vi "Convert Waveform to Data.vi"(0 "Waveform Graph":digitalwaveform(graph), 1 "Register":u8=28 format="%.0x", 2 "Ext_Read_Num_Reg":u8) -> (4 "Converted Data":T1 {"Register" max=31 format="%.0x"; "Slave Address" max=15 format="%.0x"}, 6 "Ext_Read_Reg":i32[](array[numeric]), 8 "Ext_Read_Data":u8[](array[numeric]))   [LabVIEW 2013]
uses:
  <vilib>/Waveform/DTblOps.llb/DTbl Digital to Boolean Array.vi
panel:
  # "i"
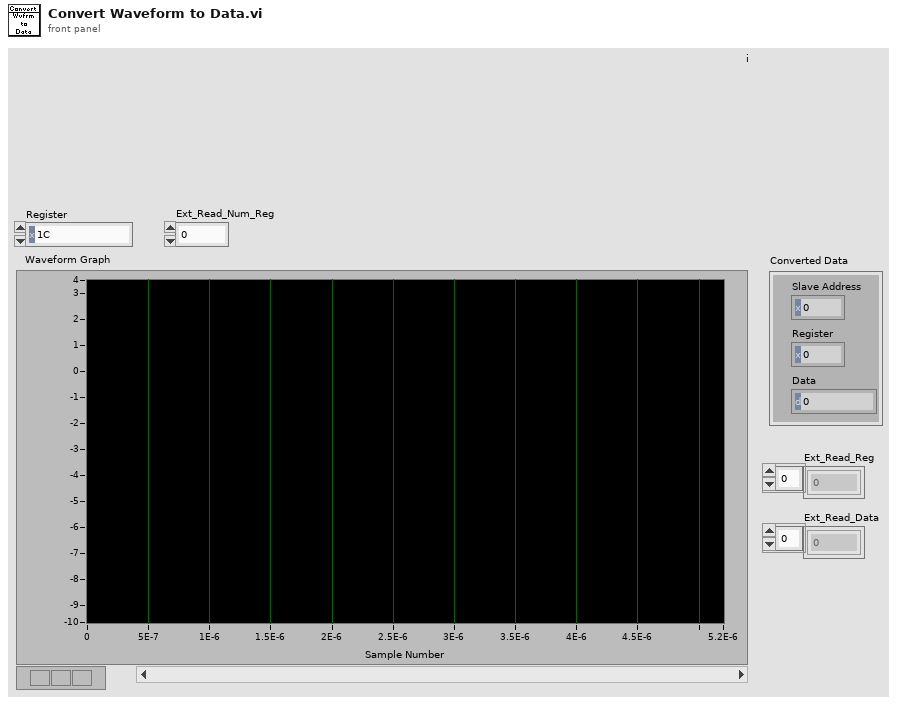
[diagram p1: front panel]
types:
  T1 = cluster{"Slave Address":u8, "Register":u8, "Data":u8}
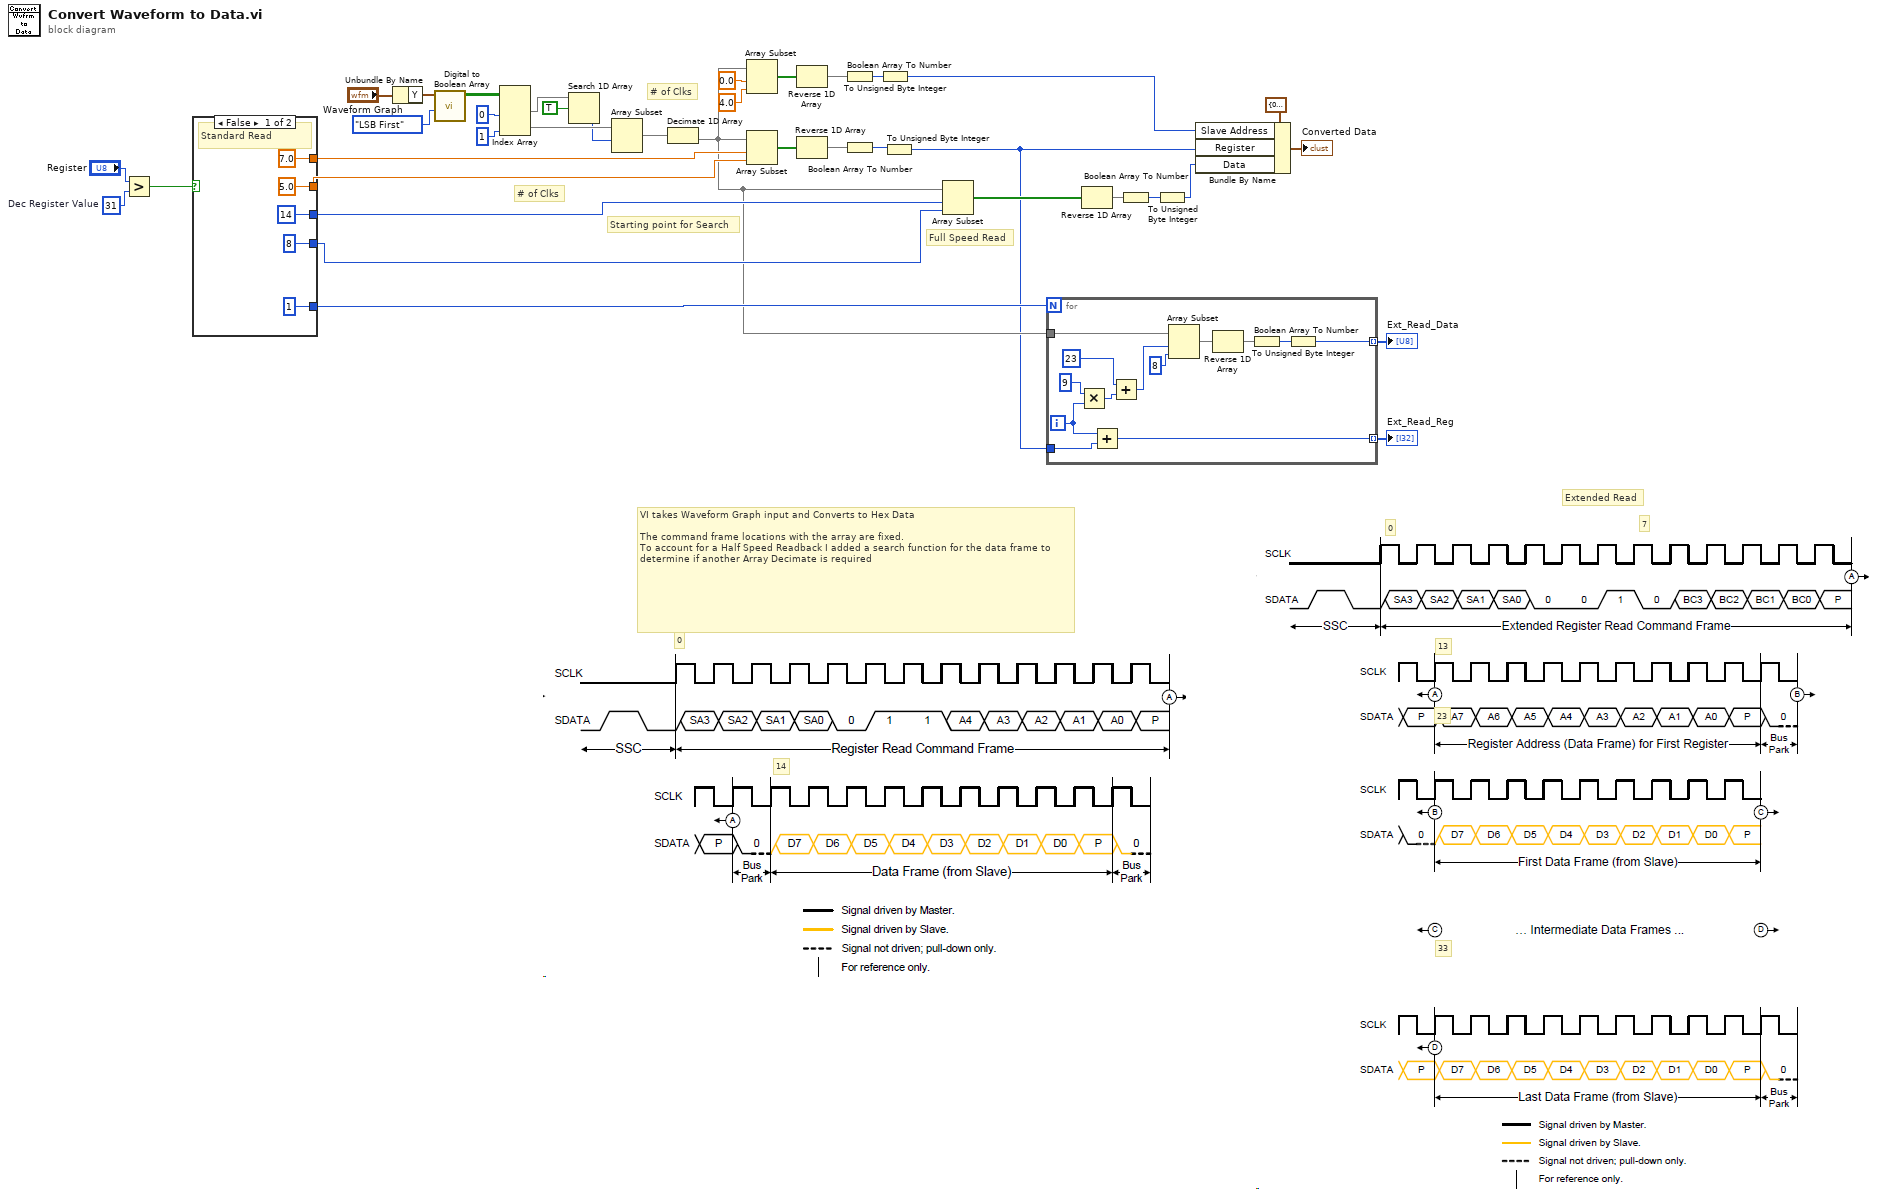
[diagram p0: block diagram]
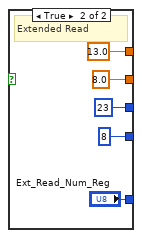
[diagram p2: hidden frame]
diagram:
  w12 = u8 31  # Dec Register Value
  # "0"
  # "0"
  # "Full Speed Read"
  # "Extended Read"
  # "33"
  # "23"
  # "13"
  # "7"
  # "Starting point for Search"
  # "# of Clks"
  # "# of Clks"
  # "VI takes Waveform Graph input and Converts to Hex Data\n\nThe command frame locations with the array are fixed.\nTo account for a Half Speed Readback I added a search function for the data frame to determine if another Array Decimate is required"
  # "14"
  n1 = Greater?(x="Register", y=w12) -> (0:w1:bool)
  n2 = case shown="False" w1 {
    tunnel: [7.0 ("input variable") 13.0 ("input variable")] -> w11
    tunnel: [5.0 ("input variable") 8.0 ("input variable")] -> w10
    tunnel: [14 ("start index (0)") 23 ("start index (0)")] -> w8
    tunnel: [8 ("length") 8 ("length")] -> w9
    tunnel: [1 ("length") "Ext_Read_Num_Reg"] -> w6
    frame False {
      # "Standard Read"
    }
    frame True {
      # "Extended Read"
    }
  }
  n3 = Unbundle By Name("Waveform Graph") -> ("Y"=w29:digitaldata)
  n4 = call-poly <vilib>:"Digital to Boolean Array.vi"("mode"=enum16{"LSB First", "MSB First"}."LSB First", "digital data"=w29) -> ("boolean array"=w36:bool[][])  [unwired: 8 in, 1 out]
  n5 = Index Array(array=w36, index (col) #1=0 ("disabled index (col)"), index (col) #2=1 ("index (col)")) -> (element #1=w28:bool[], element #2=w26:bool[])  [unwired: 2 in]
  n6 = Search 1D Array(1D array=w28, element=TRUE) -> (index of element=w7:i32)  [unwired: 1 in]
  n7 = Array Subset(array=w26, index=w7) -> (w23:bool[])  [unwired: 1 in]
  n8 = Decimate 1D Array(w23) -> (w5:bool[])  [unwired: 1 out]
  n9 = Array Subset(array=w5, index=0.0 ("input variable"), length=4.0 ("input variable")) -> (w22:bool[])
  n10 = Array Subset(array=w5, index=w11, length=w10) -> (w20:bool[])
  n11 = Reverse 1D Array(array=w22) -> (reversed array=w21:bool[])
  n12 = Reverse 1D Array(array=w20) -> (reversed array=w19:bool[])
  n13 = Boolean Array To Number(Boolean array=w21) -> (number=w33:u32)
  n14 = Boolean Array To Number(Boolean array=w19) -> (number=w18:u32)
  n15 = To Unsigned Byte Integer(number=w33) -> (unsigned 8bit integer=w30:u8)
  n16 = To Unsigned Byte Integer(number=w18) -> (unsigned 8bit integer=w4:u8)
  n17 = Array Subset(array=w5, index=w8, length=w9) -> (w14:bool[])
  n18 = for {
    N: w6 -> [_]
    tunnel: w5 -> [w58]
    tunnel: [w52] -> w3 mode=indexing
    tunnel: w4 -> [w51]
    tunnel: [w49] -> w2 mode=indexing
    i -> [w50]
    n19 = Multiply(x=9 ("start index (0)"), y=w50) -> (x*y=w55:i32)
    n20 = Add(x=w50, y=w51) -> (x+y=w49:i32)
    n21 = Add(x=23 ("start index (0)"), y=w55) -> (x+y=w53:i32)
    n22 = Array Subset(array=w58, index=w53, length=8) -> (w61:bool[])
    n23 = Reverse 1D Array(array=w61) -> (reversed array=w59:bool[])
    n24 = Boolean Array To Number(Boolean array=w59) -> (number=w60:u32)
    n25 = To Unsigned Byte Integer(number=w60) -> (unsigned 8bit integer=w52:u8)
  }
  "Ext_Read_Data" <- w3
  "Ext_Read_Reg" <- w2
  n26 = Reverse 1D Array(array=w14) -> (reversed array=w17:bool[])
  n27 = Boolean Array To Number(Boolean array=w17) -> (number=w16:u32)
  n28 = To Unsigned Byte Integer(number=w16) -> (unsigned 8bit integer=w15:u8)
  n29 = Bundle By Name(cluster=T1 {"Slave Address"=0, "Register"=0, "Data"=0} ("Write Data"), "Slave Address"=w30, "Register"=w4, "Data"=w15) -> (→"Converted Data":T1)
